vi "DFD IIR Notch Peak Design by Q.vi"(6 "fs [Hz]":dbl=1.0 format="%.2f", 7 "filter type":enum16{"Notch", "Peak"}(ring), 8 "error in (no error)":errorcluster, 10 "Q factor":dbl=20.0 format="%.2f", 11 "f0 [Hz]":dbl=0.1 format="%.2f") -> (0 "error out":errorcluster, 3 "filter out":T1={"mSRate_Fs"=1.0, "mSRate_Version"="2.0", "mSRate_Comments"="", "mSRate_OrgCoef"={"type"=enum."Undefined", "gain"=1.0, "coef a (k)"=[], "coef b (v)"=[]}, "mSRate_CurCoef"={"type"=enum."Undefined", "gain"=1.0, "coef a (k)"=[], "coef b (v)"=[]}, "mSRate_Quantized?"=FALSE, "mSRate_QCoef"={"type"=enum."Undefined", "gain"=1.0, "coef a (k)"=[], "coef b (v)"=[]}, "mSRate_QSettings"=[], "mSRate_Order"=0, "mSRate_Scaling"={"mSRate_ScaleByPowerOf2?"=FALSE, "mSRate_ScaleType"=enum."No Norm"}} {"mSRate_QSettings"."source" items=["Coef a/k"=0, "Coef b/v"=7, "Input"=1, "Output"=2, "Multiplicand"=3, "Product"=4, "Sum"=5, "Delay"=6, "Gain"=8]})   [LabVIEW 2017, in "NI_DigFilterLicensed.lvlib"]
doc: "Designs a notch or peak filter in which the notch or peak is located at the center frequency. You must manually select the polymorphic instance you want to use."
uses:
  <vilib>/addons/Digital Filter Design/NI_DigFilterLicensed.lvlib
  <vilib>/addons/Digital Filter Design/_Objects.llb/DFD Filter Obj.ctl
  <vilib>/addons/Digital Filter Design/_Objects.llb/DFD Filter Coef.ctl
  <vilib>/addons/Digital Filter Design/_Objects.llb/DFD Filter Structure Type Selector.ctl
  <vilib>/addons/Digital Filter Design/_Objects.llb/dfd_Internal Quantization Settings.ctl
  <vilib>/addons/Digital Filter Design/_Objects.llb/dfd_Internal Quantization Srcs.ctl
  <vilib>/addons/Digital Filter Design/_Objects.llb/DFD Coef Norm Type.ctl
  <vilib>/addons/Digital Filter Design/NI_DigFilter_Design.lvlib
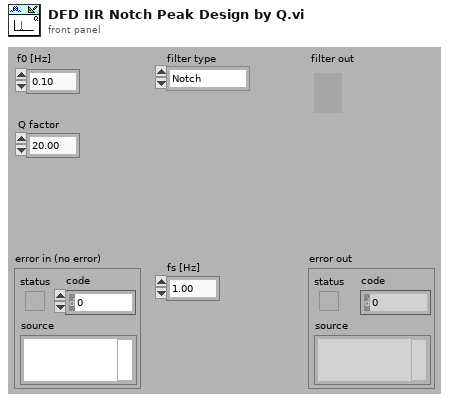
[diagram p1: front panel]
types:
  T1 = typedef "NI_DigFilterLicensed.lvlib/DFD Filter Obj.ctl" = cluster{"mSRate_Fs":dbl, "mSRate_Version":string, "mSRate_Comments":string, "mSRate_OrgCoef":T2, "mSRate_CurCoef":T2, "mSRate_Quantized?":bool, "mSRate_QCoef":T2, "mSRate_QSettings":T4[], "mSRate_Order":i32, "mSRate_Scaling":cluster{"mSRate_ScaleByPowerOf2?":bool, "mSRate_ScaleType":T6}}
  T2 = typedef "NI_DigFilterLicensed.lvlib/DFD Filter Coef.ctl" = cluster{"type":T3, "gain":dbl, "coef a (k)":dbl[], "coef b (v)":dbl[]}
  T3 = typedef "NI_DigFilterLicensed.lvlib/DFD Filter Structure Type Selector.ctl" = enum16{"Undefined", "FIR Direct Form", "FIR Direct Form Transposed", "FIR Symmetric", "FIR Antisymmetric", "IIR Direct Form I", "IIR Direct Form I Transposed", "IIR Direct Form II", "IIR Direct Form II Transposed", "IIR Cascaded Second Order Sections Form I", "IIR Cascaded Second Order Sections Form I Transposed", "IIR Cascaded Second Order Sections Form II", "IIR Cascaded Second Order Sections Form II Transposed", "Lattice Allpass (basic sections)", "Lattice Allpass (one multiplier sections)", "Lattice Allpass (normalized sections)", "Lattice AR (basic sections)", "Lattice AR (one multiplier sections)", "Lattice AR (normalized sections)", "Lattice MA (minimum phase)", "Lattice MA (maximum phase)", "Lattice ARMA (basic sections)", "Lattice ARMA (one multiplier sections)", "Lattice ARMA (normalized sections)"}
  T4 = typedef "NI_DigFilterLicensed.lvlib/dfd_Internal Quantization Settings.ctl" = cluster{"source":T5, "wl":i16, "iwl":i16, "overflow mode":enum16{"Saturation", "Wrap"}, "rounding mode":enum16{"Nearest", "Truncation"}, "signed?":bool}
  T5 = typedef "NI_DigFilterLicensed.lvlib/dfd_Internal Quantization Srcs.ctl" = u16
  T6 = typedef "NI_DigFilterLicensed.lvlib/DFD Coef Norm Type.ctl" = enum16{"No Norm", "Time Domain 1-Norm", "Time Domain 2-Norm", "Time Domain Inf-Norm"}
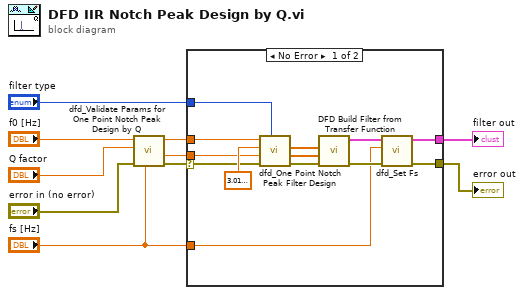
[diagram p0: block diagram]
diagram:
  n1 = call <vilib>:"dfd_Validate Params for One Point Notch Peak Design by Q.vi"("fs [Hz]"="fs [Hz]", "error in (no error)"="error in (no error)", "Q factor"="Q factor", "f0 [Hz]"="f0 [Hz]") -> ("error out"=w2:errorcluster, "normalized bandwidth"=w5:dbl, "normalized f0"=w6:dbl)  [unwired: 5 out]
  n2 = case shown="No Error" w2 {
    selector: w2 -> [w11 w23]
    tunnel: [w22 w23] -> w1
    tunnel: [w21 _] -> w10
    tunnel: "filter type" -> [w20 _]
    tunnel: w6 -> [w14 _]
    tunnel: w5 -> [w13 _]
    tunnel: "fs [Hz]" -> [w12 _]
    frame No Error {
      n3 = call <vilib>:"dfd_One Point Notch Peak Filter Design.vi"("filter type"=w20, "normalized BW"=w13, "Ab [dB]"=3.010299956639812, "normalized f0"=w14) -> ("denominator"=w16:dbl[], "numerator"=w17:dbl[])  [unwired: 2 in, 4 out]
      n4 = call <vilib>:"DFD Build Filter from Transfer Function.vi"("error in (no error)"=w11, "denominator"=w16, "numerator"=w17) -> ("error out"=w18:errorcluster, "filter out"=w19:T1)  [unwired: 1 in, 6 out]
      n5 = call <vilib>:"dfd_Set Fs.vi"("error in (no error)"=w18, "fs [Hz]"=w12, "filter in"=w19) -> ("error out"=w22:errorcluster, "filter out"=w21:T1)  [unwired: 7 out]
    }
    frame Error {
    }
  }
  "filter out" <- w10
  "error out" <- w1
